vi "AutoInstaller.vi"() -> ()   [LabVIEW 2014]
uses:
  <vilib>/zip/NI_Unzip.lvlib
panel:
  out "Text":string
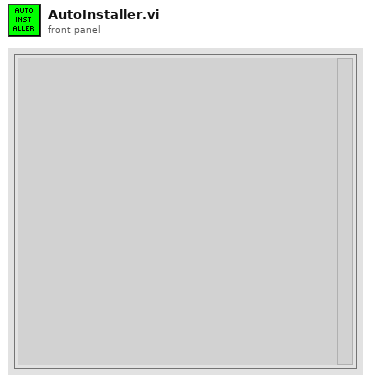
[diagram p1: front panel]
types:
  T1 = cluster{"BuildFolder":path, "Files":cluster{"ZipFile":path, "UnzippedFolder":path, "LVPath":path, "LvVer":i32, "Bit":i32}[], "LogFile":path, "pattern":string}
  T2 = cluster{"ZipFile":path, "UnzippedFolder":path, "LVPath":path, "LvVer":i32, "Bit":i32}
  T3 = cluster{"ZipFile":path, "UnzippedFolder":path, "LVPath":path, "LvVer":i32, "Bit":i32}[]
  T4 = enum32{"invalid app kind", "Development System", "Run Time System", "Student Edition", "Embedded LabVIEW", "Evaluation", "Custom"}
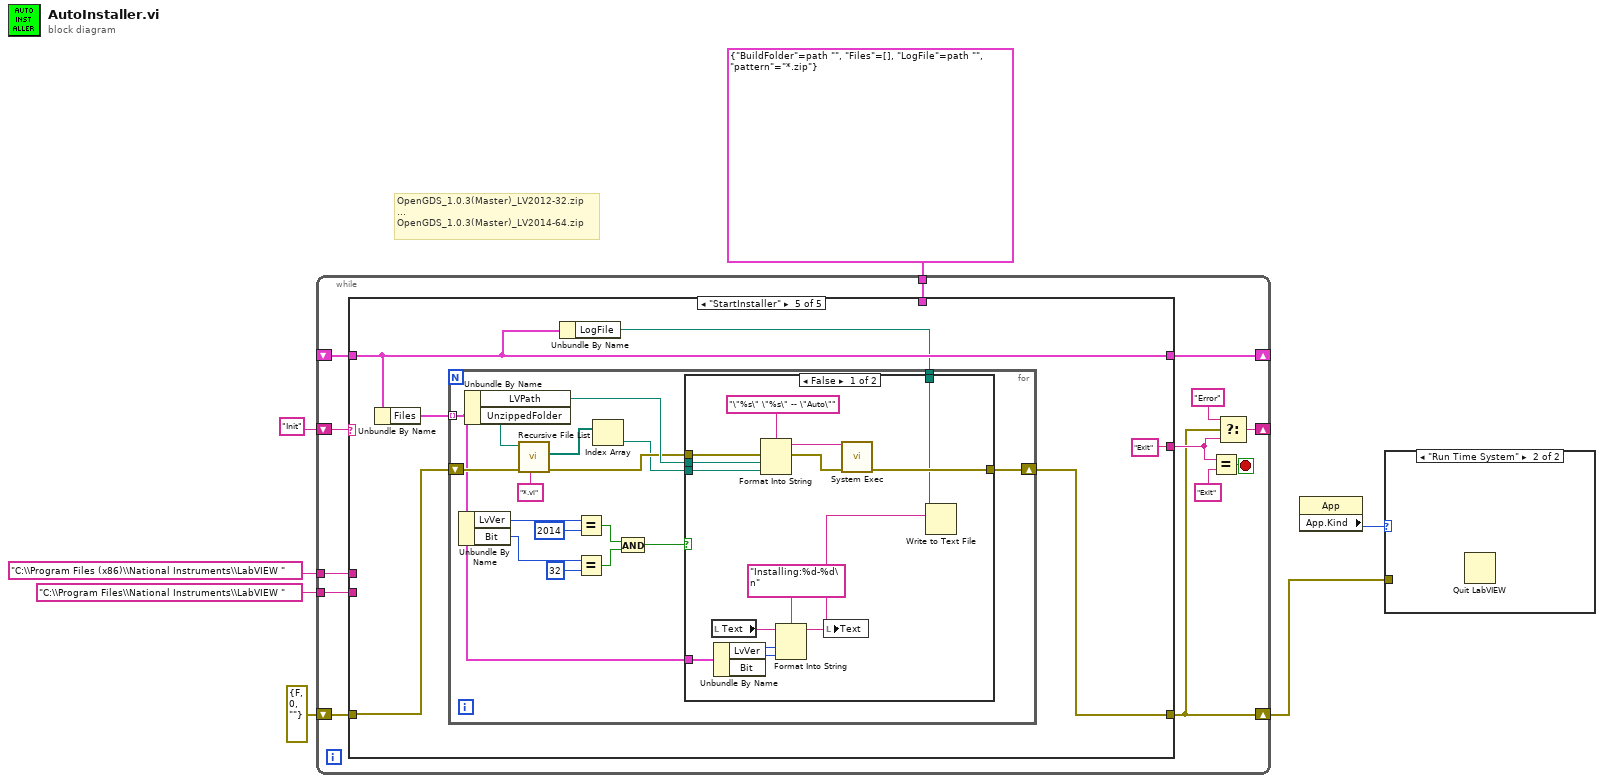
[diagram p0: block diagram]
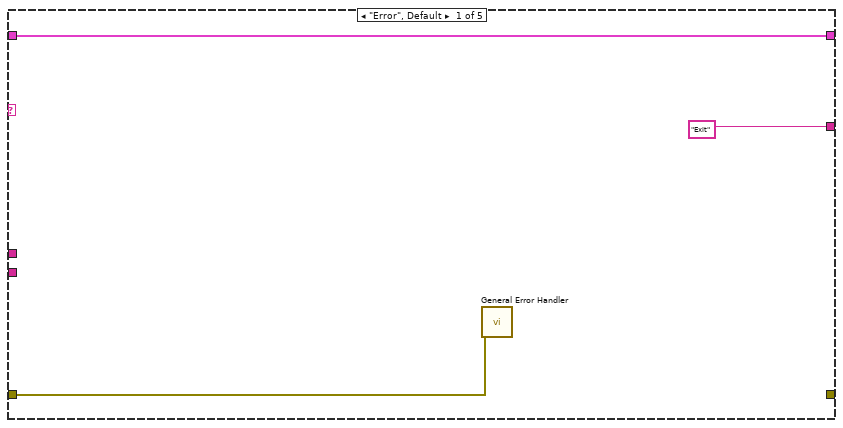
[diagram p3: hidden frame]
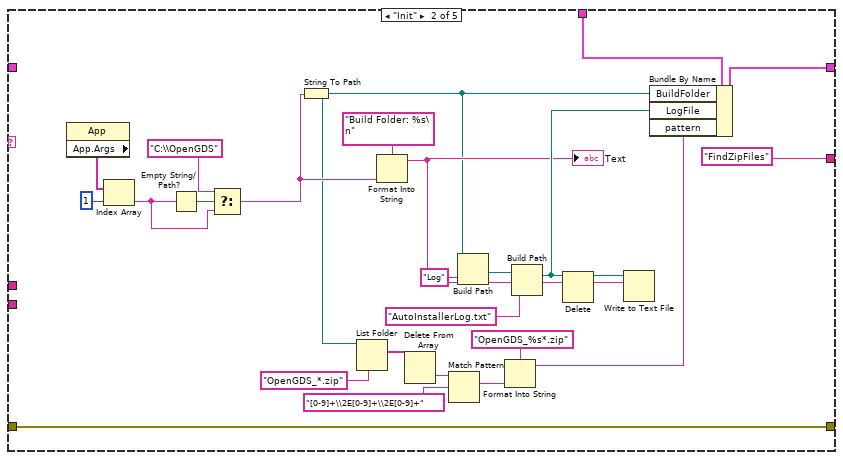
[diagram p4: hidden frame]
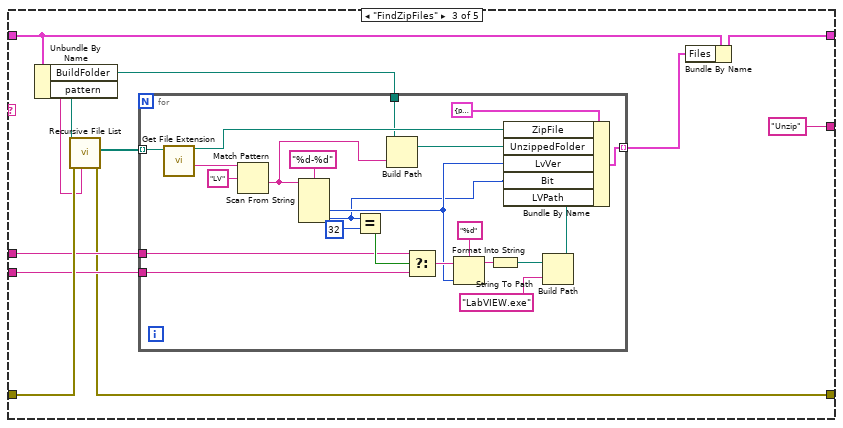
[diagram p5: hidden frame]
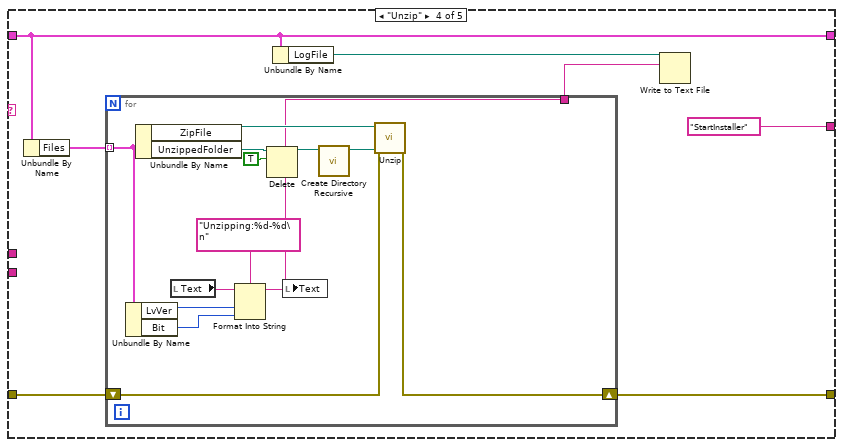
[diagram p6: hidden frame]
diagram:
  # "OpenGDS_1.0.3(Master)_LV2012-32.zip\n...\nOpenGDS_1.0.3(Master)_LV2014-64.zip"
  n1 = while {
    shift-right: [w13] -> w1
    shift-left: errorcluster {"status"=FALSE, "code"=0, "source"=""} ("error IO") -> [w20]
    shift-right: [w18] -> _
    shift-left: "Init" -> [w19]
    shift-right: [w12] -> _
    shift-left: _ -> [w11]
    tunnel: T1 {"BuildFolder"=path "", "Files"=[], "LogFile"=path "", "pattern"="*.zip"} -> [w10]
    tunnel: "C:\\Program Files (x86)\\National Instruments\\LabVIEW " -> [w9]
    tunnel: "C:\\Program Files\\National Instruments\\LabVIEW " -> [w8]
    stop <- w17 stop-if-true
    n2 = case shown="\"StartInstaller\"" w19 {
      tunnel: w20 -> [w21 w47 w56 w86 w106]
      tunnel: [_ w47 w51 w85 w104] -> w13
      tunnel: ["Exit" "FindZipFiles" "Unzip" "StartInstaller" "Exit"] -> w14
      tunnel: [w22 w46 w57 w84 w103] -> w12
      tunnel: w11 -> [w22 _ w58 w84 w103]
      tunnel: w10 -> [_ w42 _ _ _]
      tunnel: w9 -> [_ _ w54 _ _]
      tunnel: w8 -> [_ _ w53 _ _]
      frame "Error", Default {
        n3 = call <vilib>:"General Error Handler.vi"("error in (no error)"=w21) -> ()  [unwired: 10 in, 5 out]
      }
      frame "Init" {
        n4 = property class="App"() -> ("App.Args"=w43:string[])  [unwired: 2 in, 2 out]
        n5 = Index Array(array=w43, index=1) -> (element=w40:string)
        n6 = Empty String/Path?(string/path=w40) -> (empty?=w41:bool)
        n7 = Select(t="C:\\OpenGDS", s=w41, f=w40) -> (s? t:f=w39:string)
        n8 = String To Path(string=w39) -> (path=w31:path)
        n9 = List Folder(path=w31, pattern="OpenGDS_*.zip") -> (filenames=w24:string[])  [unwired: 2 in, 3 out]
        n10 = Format Into String(format string="Build Folder: %s\n", w39) -> (resulting string=w32:string)  [unwired: 2 in, 1 out]
        "Text" <- w32
        n11 = Delete From Array(array=w24) -> (deleted portion=w29:string)  [unwired: 2 in, 1 out]
        n12 = Match Pattern(string=w29, regular expression="[0-9]+\\2E[0-9]+\\2E[0-9]+") -> (match substring=w27:string)  [unwired: 1 in, 3 out]
        n13 = Build Path(base path=w31, name or relative path="Log") -> (appended path=w36:path)
        n14 = Format Into String(format string="OpenGDS_%s*.zip" ("name or relative path"), w27) -> (resulting string=w25:string)  [unwired: 2 in, 1 out]
        n15 = Build Path(base path=w36, name or relative path="AutoInstallerLog.txt") -> (appended path=w33:path)
        n16 = Delete(path (use dialog)=w33) -> (deleted path=w34:path)  [unwired: 4 in, 2 out]
        n17 = Write to Text File(file (use dialog)=w34, text=w32) -> ()  [unwired: 2 in, 3 out]
        n18 = Bundle By Name(cluster=w42, "BuildFolder"=w31, "LogFile"=w33, "pattern"=w25) -> (w46:T1)
      }
      frame "FindZipFiles" {
        n19 = Unbundle By Name(w58) -> ("BuildFolder"=w50:path, "pattern"=w49:string)
        n20 = call <vilib>:"Recursive File List.vi"("pattern"=w49, "error in (no error)"=w56, "Folder Path"=w50) -> ("error out"=w51:errorcluster, "All Files in Dir"=w55:path[])  [unwired: 4 in, 3 out]
        n21 = for {
          tunnel: w55 -> [w81] mode=indexing
          tunnel: w54 -> [w75]
          tunnel: w53 -> [w74]
          tunnel: [w64] -> w52 mode=indexing
          tunnel: w50 -> [w63]
          n22 = call <vilib>:"Get File Extension.vi"("file"=w81) -> ("filename without extension"=w80:string, "dup file"=w68:path)  [unwired: 7 in, 2 out]
          n23 = Match Pattern(string=w80, regular expression="LV") -> (after substring=w67:string)  [unwired: 1 in, 3 out]
          n24 = Scan From String(format string="%d-%d", input string=w67) -> (output 1=w61:i32, output 2=w60:i32)  [unwired: 4 in, 3 out]
          n25 = Equal?(x=w60, y=32) -> (x = y?=w76:bool)
          n26 = Build Path(base path=w63, name or relative path=w67) -> (appended path=w66:path)
          n27 = Select(t=w75, s=w76, f=w74) -> (s? t:f=w73:string)
          n28 = Format Into String(format string="%d", initial string=w73, w61) -> (resulting string=w71:string)  [unwired: 1 in, 1 out]
          n29 = String To Path(string=w71) -> (path=w70:path)
          n30 = Build Path(base path=w70, name or relative path="LabVIEW.exe") -> (appended path=w65:path)
          n31 = Bundle By Name(cluster=T2 {"ZipFile"=path "", "UnzippedFolder"=path "", "LVPath"=path "", "LvVer"=0, "Bit"=0}, "ZipFile"=w68, "UnzippedFolder"=w66, "LvVer"=w61, "Bit"=w60, "LVPath"=w65) -> (w64:T2)
        }
        n32 = Bundle By Name(cluster=w58, "Files"=w52) -> (w57:T1)
      }
      frame "Unzip" {
        n33 = Unbundle By Name(w84) -> ("Files"=w87:T3)
        n34 = for {
          tunnel: w87 -> [w92] mode=indexing
          shift-right: [w99] -> w85
          shift-left: w86 -> [w100]
          tunnel: [w89] -> w82
          n35 = Unbundle By Name(w92) -> ("LvVer"=w91:i32, "Bit"=w90:i32)
          n36 = Unbundle By Name(w92) -> ("ZipFile"=w101:path, "UnzippedFolder"=w98:path)
          n37 = local read "Text"() -> (w94:string)
          n38 = Format Into String(format string="Unzipping:%d-%d\n", initial string=w94, w91, w90) -> (resulting string=w89:string)  [unwired: 1 in, 1 out]
          n39 = Delete(path (use dialog)=w98, entire hierarchy (F)=TRUE) -> (deleted path=w96:path)  [unwired: 3 in, 2 out]
          n40 = local write "Text"(w89) -> ()
          n41 = call <vilib>:"Create Directory Recursive.vi"("directory"=w96) -> ("directory copy"=w95:path)  [unwired: 4 in, 2 out]
          n42 = call <vilib>:"Unzip.vi"("error in (no error)"=w100, "Target directory (same as Zip file if empty)"=w95, "Zip file"=w101) -> ("error out"=w99:errorcluster)  [unwired: 6 in, 2 out]
        }
        n43 = Unbundle By Name(w84) -> ("LogFile"=w83:path)
        n44 = Write to Text File(file (use dialog)=w83, text=w82) -> ()  [unwired: 2 in, 3 out]
      }
      frame "StartInstaller" {
        n45 = Unbundle By Name(w103) -> ("Files"=w107:T3)
        n46 = Unbundle By Name(w103) -> ("LogFile"=w102:path)
        n47 = for {
          tunnel: w107 -> [w109] mode=indexing
          shift-right: [w121] -> w104
          shift-left: w106 -> [w123]
          tunnel: w102 -> [w108]
          n48 = Unbundle By Name(w109) -> ("LvVer"=w116:i32, "Bit"=w113:i32)
          n49 = Unbundle By Name(w109) -> ("LVPath"=w119:path, "UnzippedFolder"=w124:path)
          n50 = call <vilib>:"Recursive File List.vi"("pattern"="*.vi", "error in (no error)"=w123, "Folder Path"=w124) -> ("error out"=w118:errorcluster, "All Files in Dir"=w120:path[])  [unwired: 4 in, 3 out]
          n51 = Equal?(x=w116, y=2014) -> (x = y?=w112:bool)
          n52 = Equal?(x=w113, y=32) -> (x = y?=w111:bool)
          n53 = Index Array(array=w120) -> (element=w117:path)  [unwired: 1 in]
          n54 = And(x=w112, y=w111) -> (x .and. y?=w110:bool)
          n55 = case shown="False" w110 {
            tunnel: [w137 w139] -> w121
            tunnel: w119 -> [w136 _]
            tunnel: w118 -> [w134 w139]
            tunnel: w117 -> [w132 _]
            tunnel: w109 -> [w127 _]
            tunnel: w108 -> [w126 _]
            frame False {
              n56 = local read "Text"() -> (w131:string)
              n57 = Unbundle By Name(w127) -> ("LvVer"=w129:i32, "Bit"=w128:i32)
              n58 = Format Into String(format string="\"%s\" \"%s\" -- \"Auto\"", error in=w134, w136, w132) -> (resulting string=w138:string, error out=w133:errorcluster)  [unwired: 1 in]
              n59 = Format Into String(format string="Installing:%d-%d\n", initial string=w131, w129, w128) -> (resulting string=w125:string)  [unwired: 1 in, 1 out]
              n60 = local write "Text"(w125) -> ()
              n61 = call <vilib>:"System Exec.vi"("error in (no error)"=w133, "command line"=w138) -> ("error out"=w137:errorcluster)  [unwired: 6 in, 3 out]
              n62 = Write to Text File(file (use dialog)=w126, text=w125) -> ()  [unwired: 2 in, 3 out]
            }
            frame True {
            }
          }
        }
      }
    }
    n63 = Equal?(x=w14, y="Exit") -> (x = y?=w17:bool)
    n64 = Select(t="Error", s=w13, f=w14) -> (s? t:f=w18:string)
  }
  n65 = property class="App"() -> ("App.Kind"=w2:T4)  [unwired: 2 in, 2 out]
  n66 = case shown="\"Run Time System\"" w2 {
    tunnel: w1 -> [_ _]
    frame Default {
    }
    frame "Run Time System" {
      n67 = Quit LabVIEW() -> ()  [unwired: 1 in]
    }
  }
